vi "Autonomous Parse.vi"(0 "File Path":path, 11 "error in":errorcluster) -> (1 "Name of Play":string, 3 "DS Message":string, 4 "Number of Commands":i32, 6 "Subsystems":string[](array[string]), 8 "Commands":string[](array[string]), 10 "Inputs":string[](array[string]), 15 "errror out":errorcluster)   [LabVIEW 2017]
uses:
  <vilib>/Utility/file.llb/Read Delimited Spreadsheet (string).vi
panel:
  out "Lines":string[](array[string])
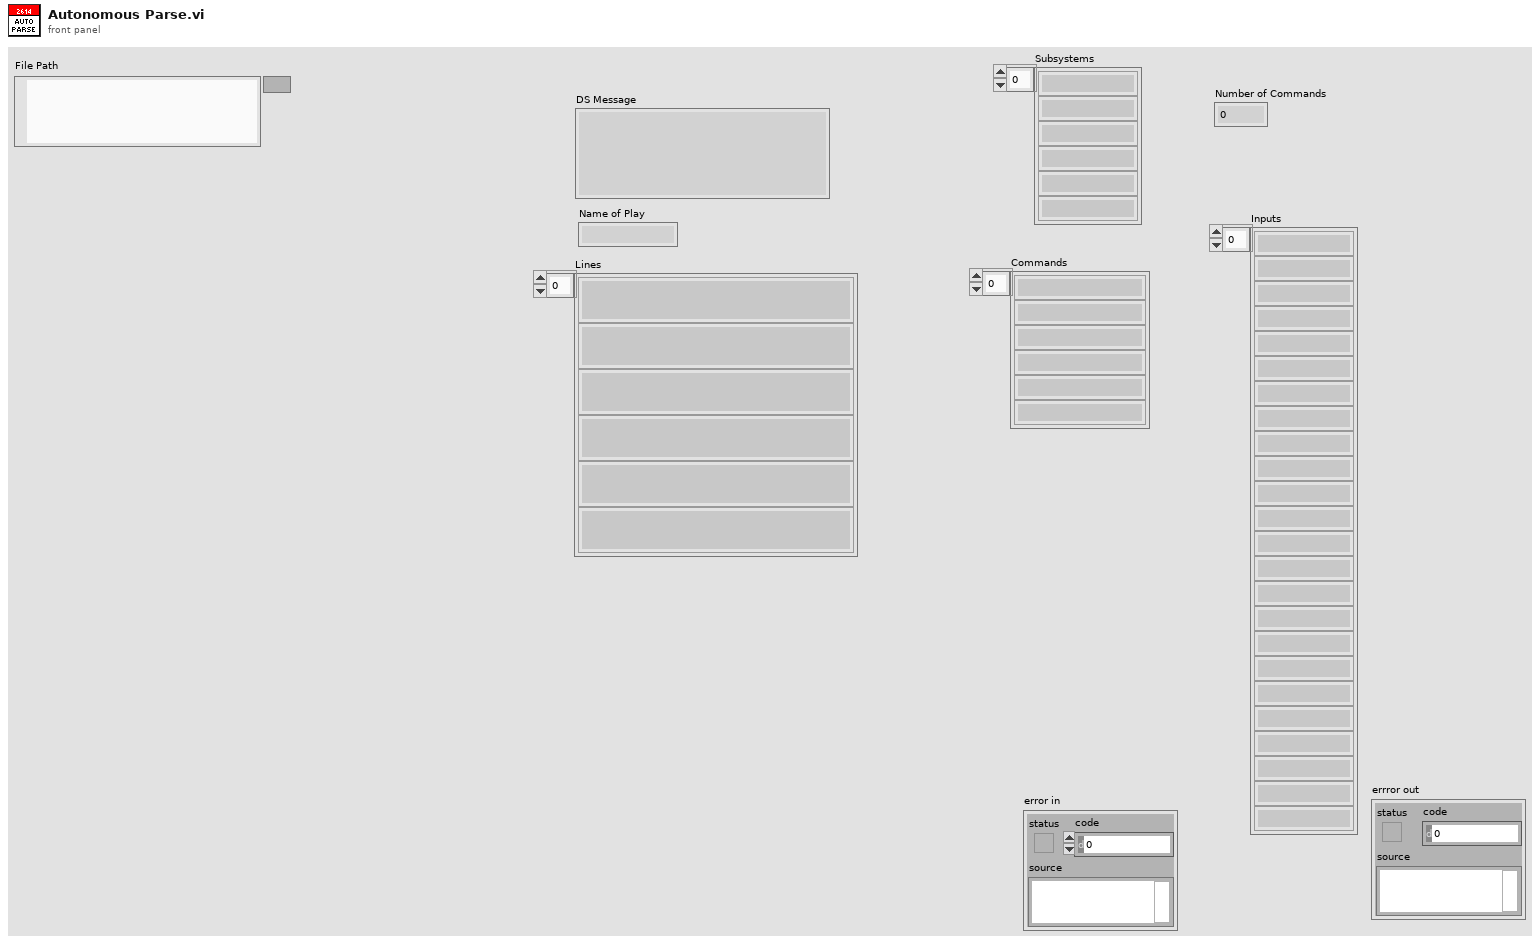
[diagram p1: front panel]
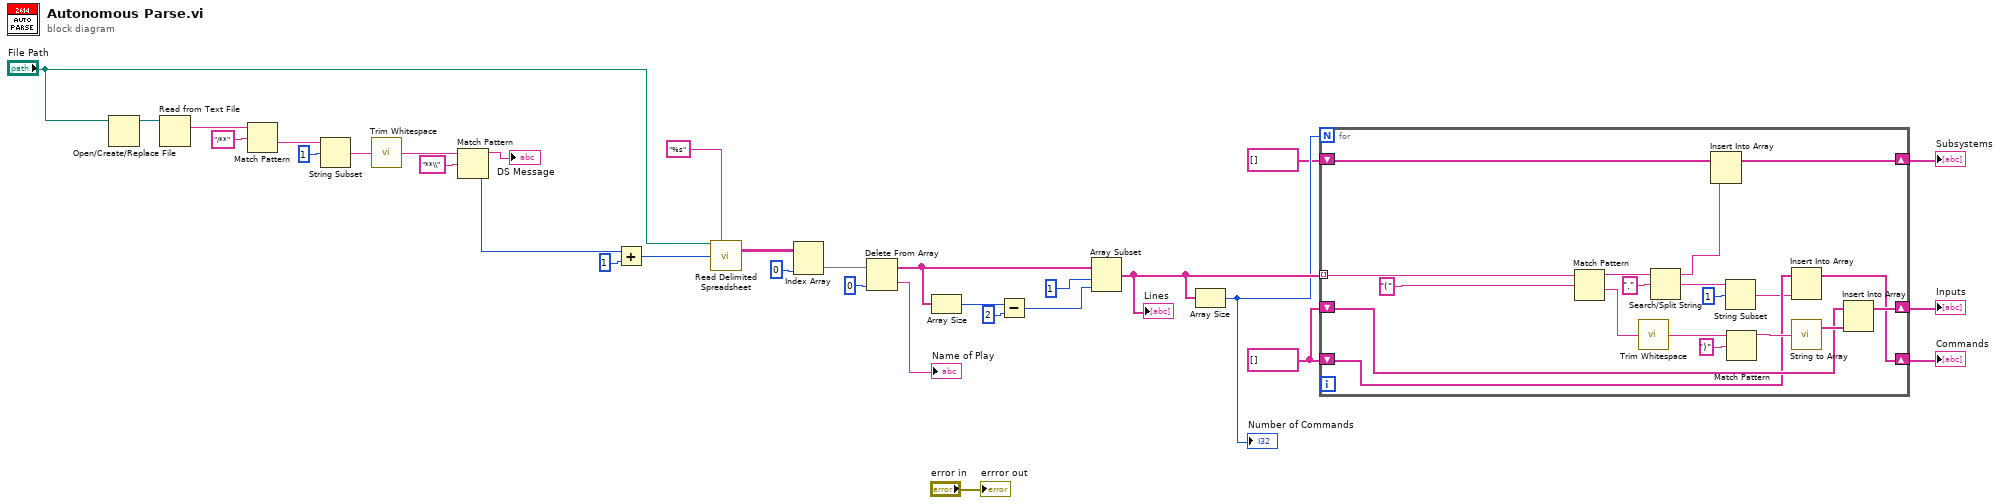
[diagram p0: block diagram]
diagram:
  w4 = string[] []
  n1 = Open/Create/Replace File(file path (use dialog)="File Path") -> (refnum out=w32:refnum<file>)  [unwired: 5 in, 2 out]
  n2 = Read from Text File(file (use dialog)=w32) -> (text=w3:string)  [unwired: 3 in, 3 out]
  n3 = Match Pattern(string=w3, regular expression="/**") -> (after substring=w30:string)  [unwired: 1 in, 3 out]
  n4 = String Subset(string=w30, offset (0)=1) -> (substring=w26:string)  [unwired: 1 in]
  n5 = call <vilib>:"Trim Whitespace.vi"("string"=w26) -> ("trimmed string"=w25:string)  [unwired: 1 in]
  n6 = Match Pattern(string=w25, regular expression="**\\") -> (before substring=→"DS Message":string, offset past match=w13:i32)  [unwired: 1 in, 2 out]
  n7 = Add(x=w13, y=1) -> (x+y=w12:i32)
  n8 = call-poly <vilib>:"Read Delimited Spreadsheet.vi"("file path (dialog if empty)"="File Path", "format (%s)"="%s", "start of read offset (chars.:0)"=w12) -> ("all rows"=w15:string[][])  [unwired: 7 in, 5 out]
  n9 = Index Array(array=w15, index (col)=0 ("disabled index (col)")) -> (element=w19:string[])  [unwired: 1 in]
  n10 = Delete From Array(array=w19, index=0) -> (deleted portion=→"Name of Play":string, array with subset deleted=w20:string[])  [unwired: 1 in]
  n11 = Array Size(array=w20) -> (size(s)=w23:i32)
  n12 = Subtract(x=w23, y=2) -> (x-y=w22:i32)
  n13 = Array Subset(array=w20, index=1, length=w22) -> (w10:string[])
  "Lines" <- w10
  n14 = Array Size(array=w10) -> (size(s)=w9:i32)
  "Number of Commands" <- w9
  n15 = for {
    N: w9 -> [_]
    tunnel: w10 -> [w46] mode=indexing
    shift-right: [w43] -> w8
    shift-left: w4 -> [w50]
    shift-right: [w42] -> w7
    shift-left: string[] [] -> [w40]
    shift-right: [w41] -> w6
    shift-left: w4 -> [w39]
    n16 = Match Pattern(string=w46, regular expression="(") -> (before substring=w37:string, after substring=w49:string)  [unwired: 1 in, 2 out]
    n17 = call <vilib>:"Trim Whitespace.vi"("string"=w49) -> ("trimmed string"=w47:string)  [unwired: 1 in]
    n18 = Search/Split String(string=w37, search string/char (-)=".") -> (substring before match=w36:string, match + rest of string=w34:string)  [unwired: 1 in, 1 out]
    n19 = Insert Into Array(array=w40, new element=w36) -> (w42:string[])  [unwired: 1 in]
    n20 = String Subset(string=w34, offset (0)=1) -> (substring=w33:string)  [unwired: 1 in]
    n21 = Match Pattern(string=w47, regular expression=")") -> (before substring=w44:string)  [unwired: 1 in, 3 out]
    n22 = Insert Into Array(array=w39, new element=w33) -> (w41:string[])  [unwired: 1 in]
    n23 = call "String to Array.vi"("Input String"=w44) -> ("Array of Strings"=w51:string[])  [unwired: 1 out]
    n24 = Insert Into Array(array=w50, new element=w51) -> (w43:string[])  [unwired: 1 in]
  }
  "Inputs" <- w8
  "Subsystems" <- w7
  "Commands" <- w6
  "errror out" <- "error in"
